vi "Get Git Tag from Path.vi"(8 "error in (no error)":errorcluster, 11 "Path":path) -> (0 "error out":errorcluster, 1 "Success?":bool, 2 "Tag":string, 3 "Repo Path":path)   [LabVIEW 2019, in "ProjectBuilder.lvlib"]
doc: "Find the tag of the Git repository that Path can be found in."
uses:
  ProjectBuilder.lvlib
  PPL/HDH.ClassLoader.lvlibp
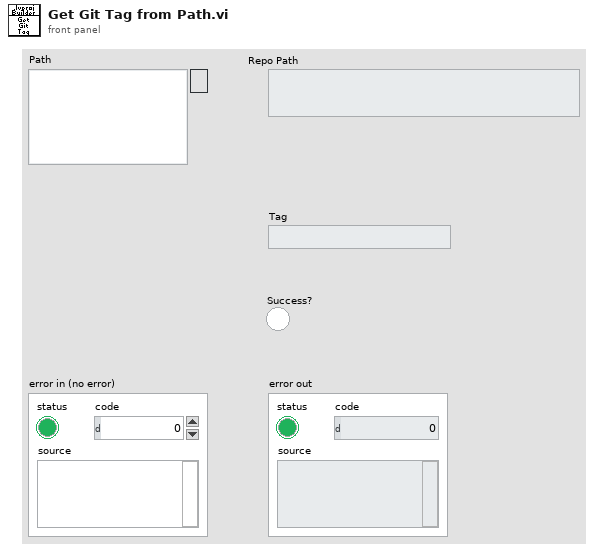
[diagram p1: front panel]
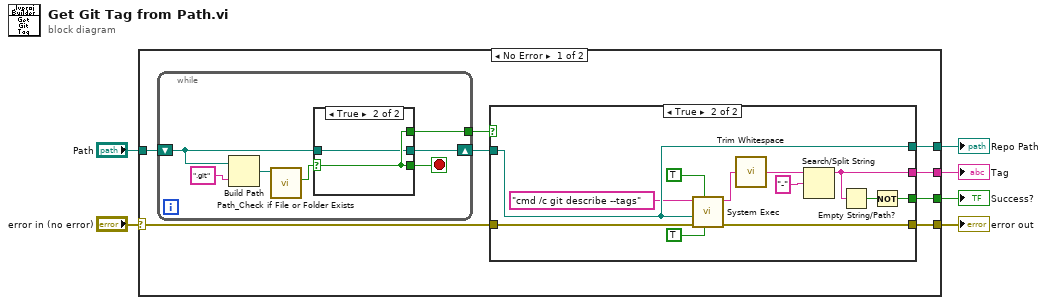
[diagram p0: block diagram]
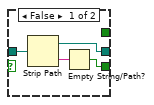
[diagram p3: hidden frame]
diagram:
  n1 = case shown="No Error" "error in (no error)" {
    selector: "error in (no error)" -> [w9 w41]
    tunnel: [w14 _] -> w6
    tunnel: [w13 _] -> w5
    tunnel: "Path" -> [w11 _]
    tunnel: [w8 w41] -> w2
    tunnel: [w7 _] -> w1
    frame No Error {
      n2 = while {
        shift-right: [w31] -> w10
        shift-left: w11 -> [w33]
        tunnel: [w30] -> w12
        stop <- w32 stop-if-true
        n3 = Build Path(base path=w33, name or relative path=".git") -> (appended path=w29:path)
        n4 = call "Path_Check if File or Folder Exists.vi"("File or Folder Path in"=w29) -> ("File or Folder Found?"=w28:bool)  [unwired: 9 in, 1 out]
        n5 = case shown="True" w28 {
          selector: w28 -> [_ w40]
          tunnel: w33 -> [w38 w39]
          tunnel: [w36 w40] -> w32
          tunnel: [w35 w39] -> w31
          tunnel: [_ w40] -> w30
          frame False {
            n6 = Strip Path(path=w38) -> (stripped path=w35:path, name=w37:string)
            n7 = Empty String/Path?(string/path=w37) -> (empty?=w36:bool)
          }
          frame True {
          }
        }
      }
      n8 = case shown="True" w12 {
        tunnel: [_ w23] -> w14
        tunnel: [_ w22] -> w13
        tunnel: w10 -> [_ w19]
        tunnel: w9 -> [w15 w21]
        tunnel: [w15 w20] -> w8
        tunnel: [_ w19] -> w7
        frame False {
        }
        frame True {
          n9 = call <vilib>:"System Exec.vi"("run minimized? (F)"=TRUE ("run minimized? (T)"), "wait until completion? (T)"=TRUE, "error in (no error)"=w21, "working directory"=w19, "command line"="cmd /c git describe --tags" ("String")) -> ("error out"=w20:errorcluster, "standard output"=w26:string)  [unwired: 3 in, 2 out]
          n10 = call <vilib>:"Trim Whitespace.vi"("string"=w26) -> ("trimmed string"=w25:string)  [unwired: 1 in]
          n11 = Search/Split String(string=w25, search string/char (-)="-") -> (substring before match=w22:string)  [unwired: 1 in, 2 out]
          n12 = Empty String/Path?(string/path=w22) -> (empty?=w24:bool)
          n13 = Not(x=w24) -> (.not. x?=w23:bool)
        }
      }
    }
    frame Error {
    }
  }
  "Success?" <- w6
  "Tag" <- w5
  "error out" <- w2
  "Repo Path" <- w1
